vi "OpenBling.vi"(4 "Mode":T1, 5 "Refresh Period (ms)":u32=500, 6 "Synchronous":bool=TRUE, 7 "Value Width":enum16{"4-bit", "8-bit"}(ring), 8 "error in (no error)":errorcluster, 9 "Chain Setup":cluster{"ChainNumber":u8, "numLeds":u8}[](array[cluster]), 10 "Reset on open?":bool, 11 "Address/COM Port":string) -> (0 "error out":errorcluster, 3 "ControlState":T2 {"ChainMask" format="0x%02x"})   [LabVIEW 2018, in "ArduinoSerialBling.lvlib"]
uses:
  ArduinoSerialBling.lvlib
  ControlState.ctl
  ConnectionType.ctl
  UdpConnection.ctl
  ChainState.ctl
  <vilib>/Instr/_visa.llb/VISA Flush IO Buffer Mask.ctl
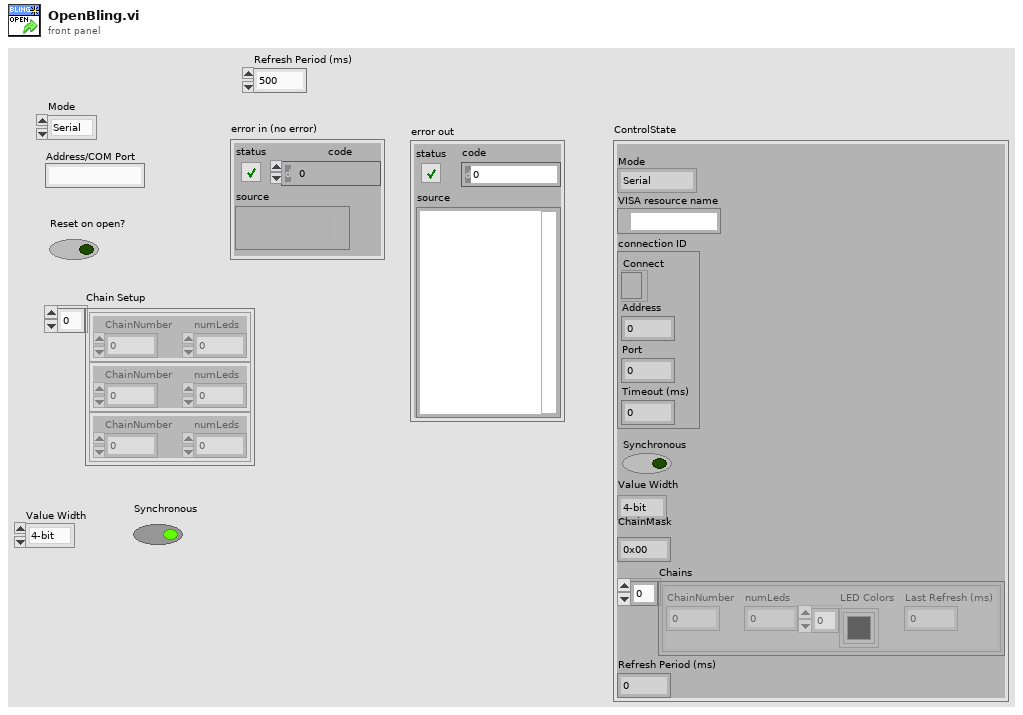
[diagram p1: front panel]
types:
  T1 = typedef "ConnectionType.ctl" = enum16{"Serial", "Ethernet", "Offline"}
  T2 = typedef "ArduinoSerialBling.lvlib/ControlState.ctl" = cluster{"Mode":T1, "VISA resource name":refnum<visa-resource-name>, "connection ID":T3, "Synchronous":bool, "Value Width":enum16{"4-bit", "8-bit"}, "ChainMask":u8, "Chains":T4[], "Refresh Period (ms)":u32}
  T3 = typedef "UdpConnection.ctl" = cluster{"Connect":refnum<k16>, "Address":u32, "Port":u16, "Timeout (ms)":i32}
  T4 = typedef "ArduinoSerialBling.lvlib/ChainState.ctl" = cluster{"ChainNumber":u8, "numLeds":u8, "LED Colors":u32[], "Last Refresh (ms)":u32}
  T5 = typedef "VISA Flush IO Buffer Mask.ctl" = u16
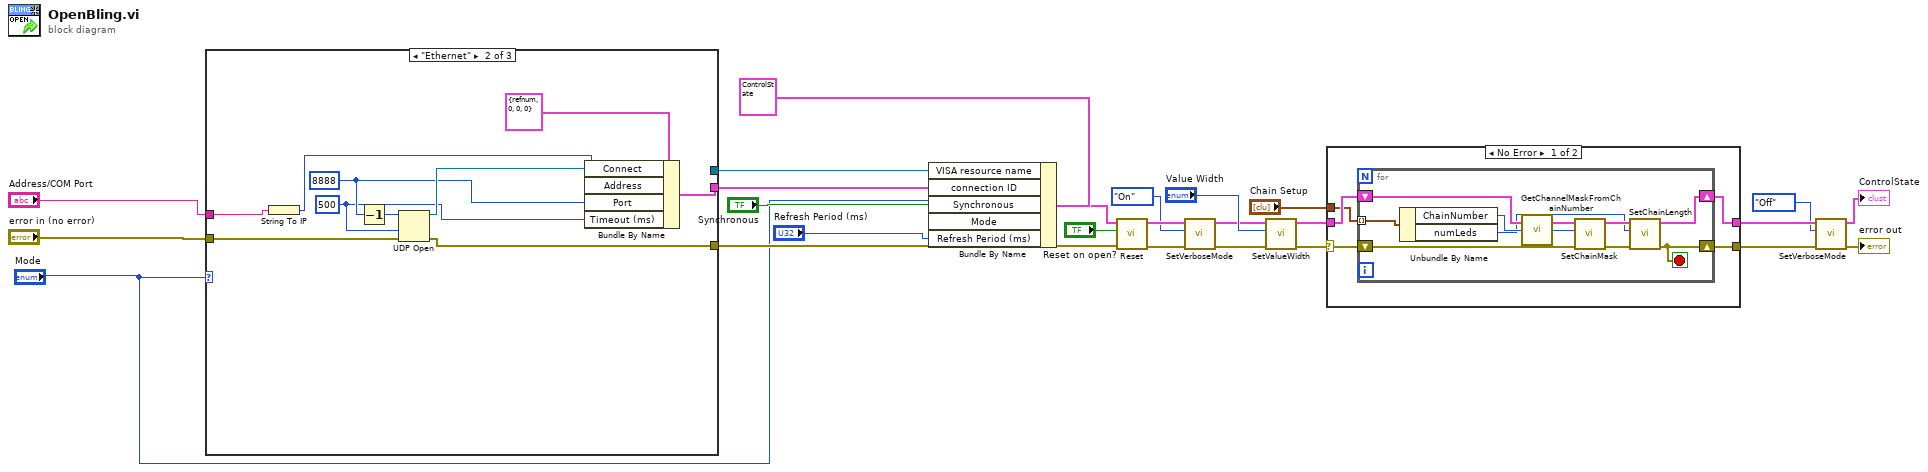
[diagram p0: block diagram]
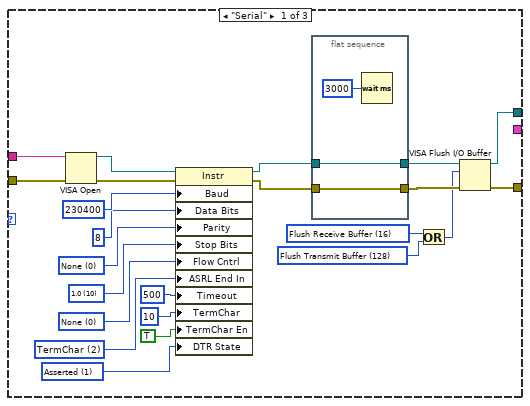
[diagram p2: hidden frame]
diagram:
  n1 = case shown="\"Ethernet\"" "Mode" {
    tunnel: [w46 _ _] -> w7
    tunnel: [w45 w59 w62] -> w6
    tunnel: "Address/COM Port" -> [w41 w61 _]
    tunnel: "error in (no error)" -> [w27 w60 w62]
    tunnel: [_ w56 _] -> w1
    frame "Serial" {
      w28 = i16 1 items=["Unknown"=-1, "Unasserted"=0, "Asserted"=1] ("Serial Settings:Modem Line Settings:Line DTR State")
      w34 = u16 2 items=["None", "Last Bit", "TermChar"] ("Serial Settings:End Mode for Reads")
      w35 = u16 0 items=["None", "XON/XOFF", "RTS/CTS", "XON/XOFF & RTS/CTS", "DTR/DSR", "XON/XOFF & DTR/DSR"] ("Serial Settings:Flow Control")
      w36 = u16 10 items=["1.0"=10, "1.5"=15, "2.0"=20] ("Serial Settings:Stop Bits")
      w37 = u16 0 items=["None", "Odd", "Even", "Mark", "Space"] ("Serial Settings:Parity")
      w42 = T5 128 items=["Flush Receive Buffer"=16, "Write Transmit Buffer to Device"=32, "Flush Receive Buffer (No I/O)"=64, "Flush Transmit Buffer"=128] ("y")
      w44 = T5 16 items=["Flush Receive Buffer"=16, "Write Transmit Buffer to Device"=32, "Flush Receive Buffer (No I/O)"=64, "Flush Transmit Buffer"=128] ("Mask")
      n2 = VISA Open(error in (no error)=w27, VISA resource name=w41) -> (VISA resource name=w40:refnum<visa-resource-name>, error out=w26:errorcluster)  [unwired: 3 in]
      n3 = property class="Instr"(reference=w40, error in=w26, "Baud"=u32 230400 ("baud rate (9600)"), "Data Bits"=u16 8 ("Serial Settings:Data Bits"), "Parity"=w37, "Stop Bits"=w36, "Flow Cntrl"=w35, "ASRL End In"=w34, "Timeout"=u32 500 ("timeout (10sec)"), "TermChar"=u8 10 ("Message Based Settings:Termination Character"), "TermChar En"=TRUE ("Message Based Settings:Termination Character Enable"), "DTR State"=w28) -> (reference out=w30:refnum<visa-resource-name>, error out=w29:errorcluster)
      n4 = flat-sequence {
        tunnel: [w51] -> w47
        tunnel: w29 -> [w51]
        tunnel: [w50] -> w48
        tunnel: w30 -> [w50]
        frame #0 {
          n5 = Wait (ms)(milliseconds to wait=u32 3000) -> ()  [unwired: 1 out]
        }
      }
      n6 = Or(x=w44, y=w42) -> (x .or. y?=w43:T5)
      n7 = VISA Flush I/O Buffer(VISA resource name=w48, mask (16)=w43, error in (no error)=w47) -> (VISA resource name out=w46:refnum<visa-resource-name>, error out=w45:errorcluster)
    }
    frame "Ethernet" {
      w53 = 500 ("timeout ms (25000)")
      w54 = u16 8888 ("port")
      n8 = String To IP(1:w61) -> (0:w55:u32)
      n9 = Decrement(x=w54) -> (x-1=w52:u16)
      n10 = UDP Open(8:w60, 9:w53, 11:w52) -> (port=w57:refnum<k16>, 0:w59:errorcluster)  [unwired: 2 in, 1 out]
      n11 = Bundle By Name(cluster=T3 {"Connect"=refnum, "Address"=0, "Port"=0, "Timeout (ms)"=0}, "Connect"=w57, "Address"=w55, "Port"=w54, "Timeout (ms)"=w53) -> (w56:T3)
    }
    frame "Offline", Default {
    }
  }
  n12 = Bundle By Name(cluster=T2 {"Mode"=enum."Serial", "VISA resource name"="", "connection ID"={"Connect"=refnum, "Address"=0, "Port"=0, "Timeout (ms)"=0}, "Synchronous"=FALSE, "Value Width"=enum."4-bit", "ChainMask"=0, "Chains"=[], "Refresh Period (ms)"=0} ("ControlState"), "VISA resource name"=w7, "connection ID"=w1, "Synchronous"="Synchronous", "Mode"="Mode", "Refresh Period (ms)"="Refresh Period (ms)") -> (w23:T2)
  n13 = call "Reset.vi"("error in (no error)"=w6, "Reset"="Reset on open?", "ControlState in"=w23) -> ("error out"=w17:errorcluster, "ControlState out"=w18:T2)  [unwired: 7 in]
  n14 = call "SetVerboseMode.vi"("error in (no error)"=w17, "Verbosity"=enum16{"Off", "On"}."On", "ControlState in"=w18) -> ("error out"=w16:errorcluster, "ControlState out"=w14:T2)  [unwired: 7 in]
  n15 = call "SetValueWidth.vi"("error in (no error)"=w16, "Value Width"="Value Width", "ControlState in"=w14) -> ("error out"=w21:errorcluster, "ControlState out"=w20:T2)  [unwired: 7 in]
  n16 = case shown="No Error" w21 {
    selector: w21 -> [w67 w78]
    tunnel: w20 -> [w66 w79]
    tunnel: "Chain Setup" -> [w65 _]
    tunnel: [w64 w79] -> w13
    tunnel: [w63 w78] -> w12
    frame No Error {
      n17 = for {
        tunnel: w65 -> [w75] mode=indexing
        shift-right: [w68] -> w64
        shift-left: w66 -> [w77]
        shift-right: [w69] -> w63
        shift-left: w67 -> [w73]
        stop <- w69 stop-if-true
        n18 = Unbundle By Name(w75) -> ("ChainNumber"=w74:u8, "numLeds"=w71:u8)
        n19 = call "GetChannelMaskFromChainNumber.vi"("ChainNumber"=w74) -> ("ChainMask"=w76:u8)
        n20 = call "SetChainMask.vi"("error in (no error)"=w73, "ChainMask"=w76, "ControlState in"=w77) -> ("error out"=w70:errorcluster, "ControlState out"=w72:T2)  [unwired: 7 in]
        n21 = call "SetChainLength.vi"("error in (no error)"=w70, "Chain Length"=w71, "ControlState in"=w72) -> ("error out"=w69:errorcluster, "ControlState out"=w68:T2)  [unwired: 7 in]
      }
    }
    frame Error {
    }
  }
  n22 = call "SetVerboseMode.vi"("error in (no error)"=w12, "Verbosity"=enum16{"Off", "On"}."Off", "ControlState in"=w13) -> ("error out"=→"error out":errorcluster, "ControlState out"=→"ControlState":T2)  [unwired: 7 in]
